vi "File.Check if File or Folder Exists.vi"(8 "error in":errorcluster, 10 "Create Dir if does not Exist":bool, 11 "Path":path) -> (0 "error out":errorcluster, 1 "Created":bool, 2 "Exists":bool, 3 "Dup Path":path, 5 "IsDir":bool)   [LabVIEW 2024, in "EQMF.lvlib" / "File Utils.lvlib"]
uses:
  File Utils.lvlib
  Status/Status Utils.lvlib
panel:
  out "Check_Exists":bool
  out "Not a Path":bool
  out "Empty":bool
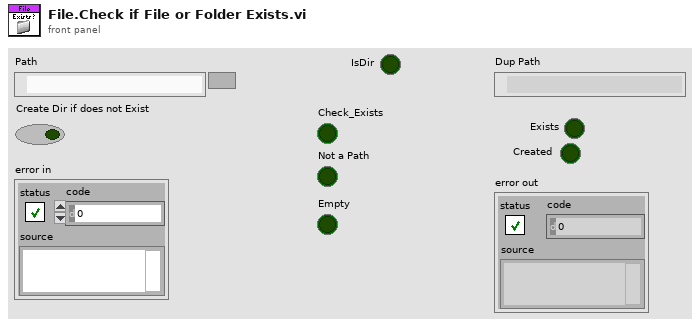
[diagram p1: front panel]
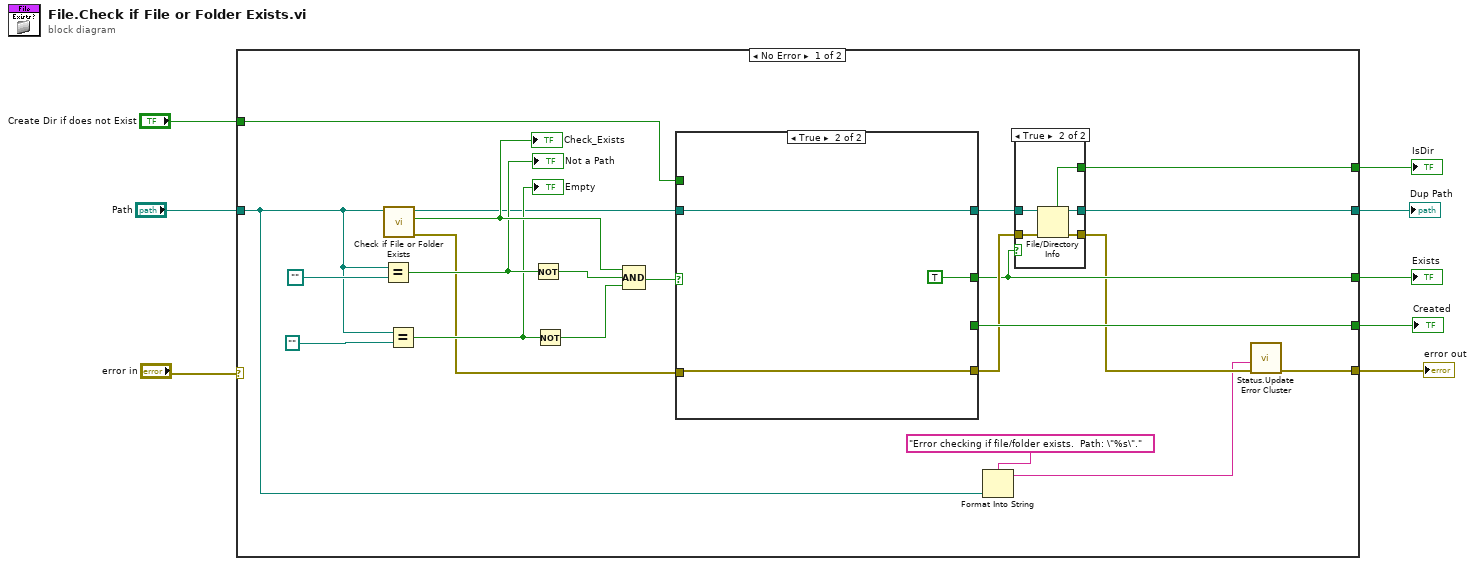
[diagram p0: block diagram]
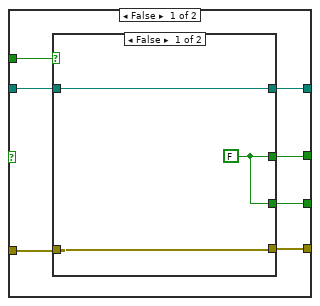
[diagram p3: hidden frame]
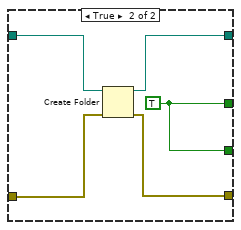
[diagram p4: hidden frame]
diagram:
  n1 = case shown="No Error" "error in" {
    selector: "error in" -> [_ w57]
    tunnel: "Path" -> [w9 w56]
    tunnel: [w15 _] -> w7
    tunnel: [w12 w57] -> w5
    tunnel: [w17 w56] -> w4
    tunnel: [w21 _] -> w3
    tunnel: "Create Dir if does not Exist" -> [w19 _]
    tunnel: [w14 _] -> w1
    frame No Error {
      n2 = Equal?(x=w9, y=path "") -> (x = y?=w28:bool)
      "Not a Path" <- w28
      n3 = call <vilib>:"Check if File or Folder Exists.vi"("path"=w9) -> ("error out"=w23:errorcluster, "file or folder exists?"=w29:bool, "dup path"=w22:path)  [unwired: 8 in]
      "Check_Exists" <- w29
      n4 = Equal?(x=w9, y=path "") -> (x = y?=w27:bool)
      "Empty" <- w27
      n5 = Not(x=w28) -> (.not. x?=w26:bool)
      n6 = Not(x=w27) -> (.not. x?=w25:bool)
      n7 = Compound Arithmetic op=AND(w29, w26, w25) -> (w20:bool)
      n8 = case shown="True" w20 {
        tunnel: w22 -> [w44 w54]
        tunnel: w23 -> [w43 w53]
        tunnel: [w42 w53] -> w16
        tunnel: [w41 w54] -> w18
        tunnel: [w38 _] -> w21
        tunnel: [w39 TRUE] -> w15
        tunnel: w19 -> [w40 _]
        frame False {
          n9 = case shown="False" w40 {
            tunnel: w44 -> [w47 w52]
            tunnel: w43 -> [w46 w51]
            tunnel: [w46 w50] -> w42
            tunnel: [w47 w49] -> w41
            tunnel: [w45 w48] -> w39
            tunnel: [w45 w48] -> w38
            frame False {
              w45 = FALSE
            }
            frame True {
              w48 = TRUE
              n10 = Create Folder(path (use dialog)=w52, error in=w51) -> (created path=w49:path, error out=w50:errorcluster)  [unwired: 1 in, 1 out]
            }
          }
        }
        frame True {
        }
      }
      n11 = Format Into String(format string="Error checking if file/folder exists.  Path: \"%s\".", w9) -> (resulting string=w11:string)  [unwired: 2 in, 1 out]
      n12 = case shown="True" w15 {
        tunnel: w18 -> [w31 w37]
        tunnel: [w31 w36] -> w17
        tunnel: [w32 w35] -> w13
        tunnel: w16 -> [w32 w34]
        tunnel: [_ w33] -> w14
        frame False {
        }
        frame True {
          n13 = File/Directory Info(path=w37, error in=w34) -> (path out=w36:path, directory=w33:bool, error out=w35:errorcluster)  [unwired: 4 out]
        }
      }
      n14 = call "Status.Update Error Cluster.vi"("Error In"=w13, "NewDesc"=w11) -> ("Error Out"=w12:errorcluster)  [unwired: 9 in]
    }
    frame Error {
    }
  }
  "Exists" <- w7
  "error out" <- w5
  "Dup Path" <- w4
  "Created" <- w3
  "IsDir" <- w1
